vi "getOffsets.vi"(8 "error in (no error)":errorcluster, 11 "Port":refnum<visa-resource-name>) -> (0 "error out":errorcluster, 3 "Port out":refnum<visa-resource-name>)   [LabVIEW 2018]
uses:
  Strict Type Controls/Settings Operation.ctl
  classes/Variable Manager/VariableManager_Bool.vi
panel:
  out "offsets Out":string[][](array[string])
  out "Array":dbl[](array[numeric])
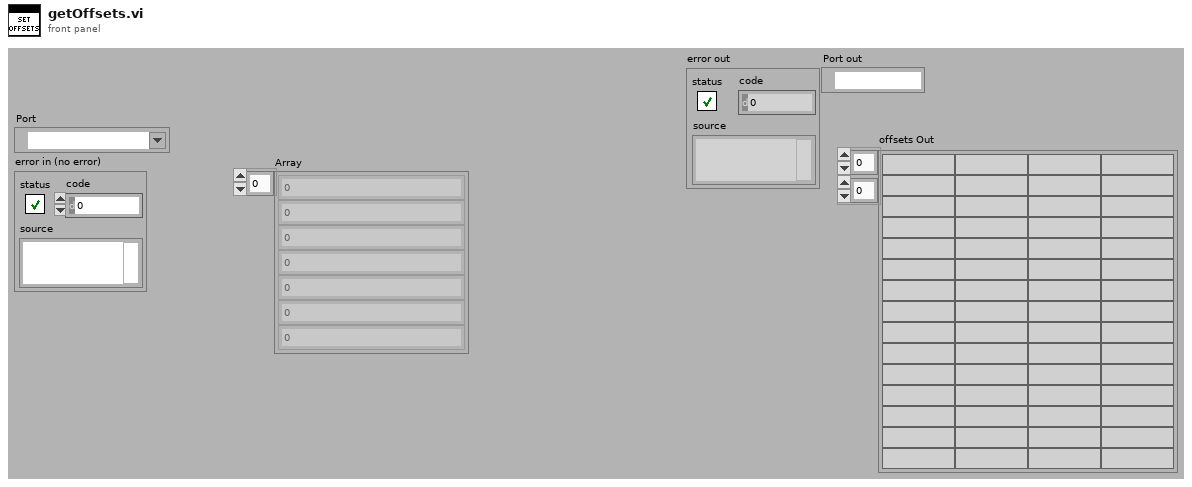
[diagram p1: front panel]
types:
  T1 = typedef "Settings Operation.ctl" = enum8{"Get Value", "Set Value", "Read File", "Write File", "Write Stored Value"}
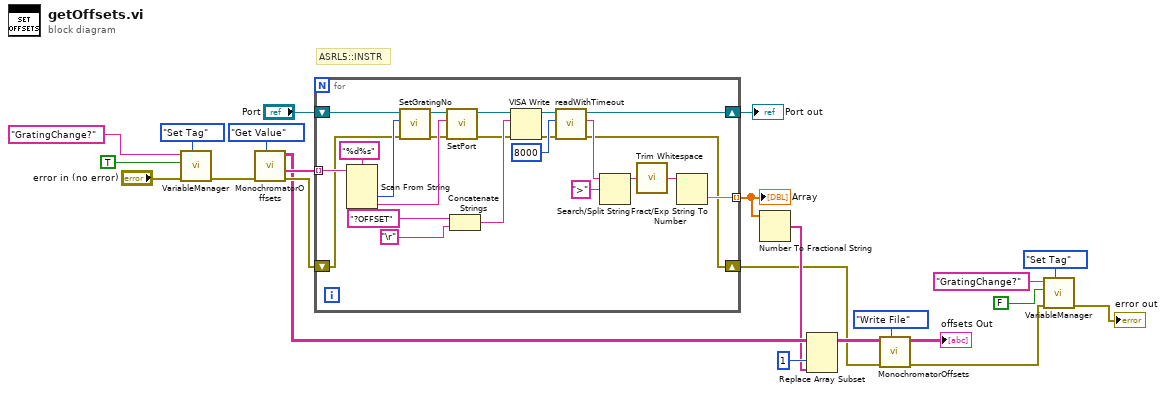
[diagram p0: block diagram]
diagram:
  # "ASRL5::INSTR"
  n1 = call-poly "VariableManager.vi"("Operation"=enum16{"Get Tag", "Set Tag"}."Set Tag", "error in (no error)"="error in (no error)", "Value"=TRUE, "Tag"="GratingChange?") -> ("error out"=w8:errorcluster)  [unwired: 4 in, 3 out]
  n2 = call "MonochromatorOffsets.vi"("Operation"=Settings_Operation."Get Value", "error in (no error)"=w8) -> ("error out"=w21:errorcluster, "Channel"=w23:string[], "offsets Out"=w20:string[][])  [unwired: 6 in, 1 out]
  n3 = for {
    tunnel: w23 -> [w46] mode=indexing
    shift-right: [w34] -> w12
    shift-left: "Port" -> [w41]
    tunnel: [w31] -> w15 mode=indexing
    shift-right: [w24] -> w4
    shift-left: w21 -> [w25]
    n4 = Scan From String(format string="%d%s", input string=w46) -> (output 1=w44:i32, output 2=w43:string)  [unwired: 4 in, 3 out]
    n5 = call "SetGratingNo.vi"("error in"=w25, "GratingNo"=w44, "Port"=w41) -> ("error out"=w27:errorcluster, "Port out"=w42:refnum<visa-resource-name>)  [unwired: 6 in, 1 out]
    n6 = call "SetPort.vi"("error in"=w27, "Slit"=w43, "Port"=w42) -> ("error out"=w26:errorcluster, "Port out"=w39:refnum<visa-resource-name>)  [unwired: 6 in, 1 out]
    n7 = Concatenate Strings("?OFFSET" ("concatenated string"), "\r") -> (w38:string)
    n8 = VISA Write(VISA resource name=w39, write buffer=w38, error in (no error)=w26) -> (VISA resource name out=w35:refnum<visa-resource-name>, error out=w33:errorcluster)  [unwired: 1 out]
    n9 = call "readWithTimeout.vi"("error in"=w33, "timeOut"=u32 8000, "Port"=w35) -> ("error out"=w24:errorcluster, "String"=w30:string, "Port out"=w34:refnum<visa-resource-name>)  [unwired: 6 in]
    n10 = Search/Split String(string=w30, search string/char (-)=">") -> (substring before match=w29:string)  [unwired: 1 in, 2 out]
    n11 = call <vilib>:"Trim Whitespace.vi"("string"=w29) -> ("trimmed string"=w28:string)  [unwired: 1 in]
    n12 = Fract/Exp String To Number(string=w28) -> (number=w31:dbl)  [unwired: 3 in, 1 out]
  }
  "Array" <- w15
  "Port out" <- w12
  n13 = Number To Fractional String(number=w15) -> (F-format string=w14:string[])  [unwired: 3 in]
  n14 = Replace Array Subset(array=w20, new element=w14, index (col)=1 ("disabled index (col)")) -> (w19:string[][])  [unwired: 1 in]
  n15 = call "MonochromatorOffsets.vi"("Operation"=Settings_Operation."Write File", "error in (no error)"=w4, "offsetsIn"=w19) -> ("error out"=w2:errorcluster, "offsets Out"=→"offsets Out":string[][])  [unwired: 5 in, 2 out]
  n16 = call-poly "VariableManager.vi"("Operation"=enum16{"Get Tag", "Set Tag"}."Set Tag", "error in (no error)"=w2, "Value"=FALSE, "Tag"="GratingChange?") -> ("error out"=→"error out":errorcluster)  [unwired: 4 in, 3 out]
